vi "DataToVAttrbutes.vi"(6 "to lowercase?(T)":bool=TRUE, 8 "error in (no error)":errorcluster, 11 "data":variant) -> (0 "error out":errorcluster, 3 "VAttributes":variant)   [LabVIEW 2019]
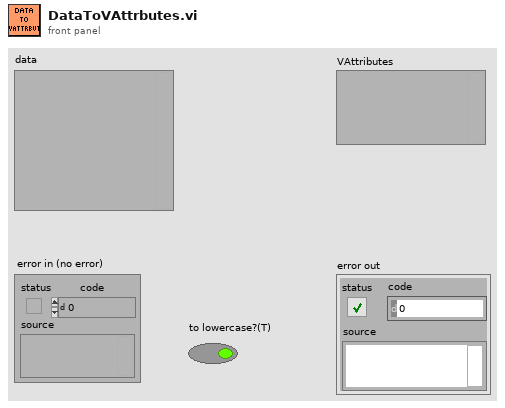
[diagram p1: front panel]
types:
  T1 = typedef "Type Descriptor Enumeration__ogtk.ctl" = enum8{"<Null>", "I8", "I16", "I32", "I64", "U8", "U16", "U32", "U64", "SGL", "DBL", "EXT", "CSG", "CDB", "CXT", "0x0F", "0x10", "0x11", "0x12", "0x13", "0x14", "Enum U8", "Enum U16", "Enum U32", "Enum U64", "SGL PQ", "DBL PQ", "EXT PQ", "CSG PQ", "CDB PQ", "CXT PQ", "0x1F", "0x20", "Boolean", "0x22", "0x23", "0x24", "0x25", "0x26", "0x27", "0x28", "0x29", "0x2A", "0x2B", "0x2C", "0x2D", "0x2E", "0x2F", "String", "0x31", "Path", "Pict", "0x34", "0x35", "0x36", "DAQ", "0x38", "0x39", "0x3A", "0x3B", "0x3C", "0x3D", "0x3E", "0x3F", "Array", "0x41", "0x42", "0x43", "0x44", "0x45", "0x46", "0x47", "0x48", "0x49", "0x4A", "0x4B", "0x4C", "0x4D", "0x4E", "0x4F", "Cluster", "0x51", "0x52", "Variant", "Waveform", "0x55", "0x56", "0x57", "0x58", "0x59", "0x5A", "0x5B", "0x5C", "0x5D", "0x5E", "0x5F", "0x60", "0x61", "0x62", "0x63", "0x64", "0x65", "0x66", "0x67", "0x68", "0x69", "0x6A", "0x6B", "0x6C", "0x6D", "0x6E", "0x6F", "Refnum"}
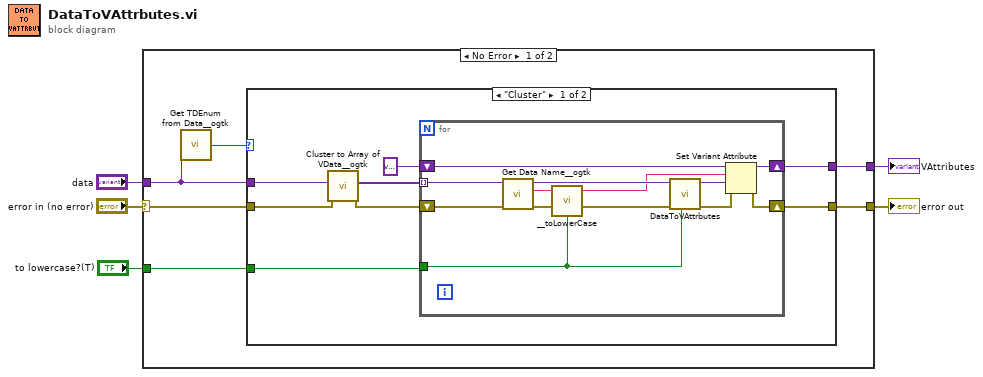
[diagram p0: block diagram]
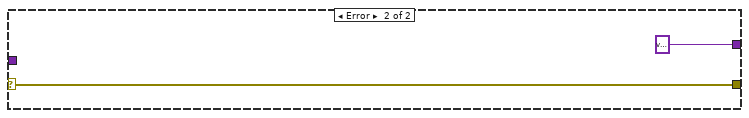
[diagram p3: hidden frame]
diagram:
  n1 = case shown="No Error" "error in (no error)" {
    selector: "error in (no error)" -> [w8 w35]
    tunnel: "data" -> [w11 _]
    tunnel: [w10 variant ("variant")] -> w4
    tunnel: [w9 w35] -> w3
    tunnel: "to lowercase?(T)" -> [w7 _]
    frame No Error {
      n2 = call <userlib>:"Get TDEnum from Data__ogtk.vi"("Data"=w11) -> ("Type Descriptor Enumeration"=w6:T1)  [unwired: 4 in]
      n3 = case shown="\"Cluster\"" w6 {
        tunnel: w11 -> [w19 w32]
        tunnel: [w18 w32] -> w10
        tunnel: [w17 w33] -> w9
        tunnel: w8 -> [w16 w33]
        tunnel: w7 -> [w15 _]
        frame "Cluster" {
          n4 = call <userlib>:"Cluster to Array of VData__ogtk.vi"("error in (no error)"=w16, "Cluster"=w19) -> ("error out"=w12:errorcluster, "Array of VData"=w14:variant[])  [unwired: 8 in]
          n5 = for {
            tunnel: w14 -> [w31] mode=indexing
            shift-right: [w28] -> w18
            shift-left: variant ("variant") -> [w29]
            shift-right: [w22] -> w17
            shift-left: w12 -> [w23]
            tunnel: w15 -> [w20]
            n6 = call <userlib>:"Get Data Name__ogtk.vi"("error in (no error)"=w23, "Data"=w31) -> ("error out"=w24:errorcluster, "Data Name"=w30:string, "Data dup"=w27:variant)  [unwired: 7 in]
            n7 = call "__toLowerCase.vi"("Data Name in"=w30, "to lowercase?(F)"=w20) -> ("Data Name out"=w21:string)  [unwired: 5 in]
            n8 = call "DataToVAttrbutes.vi"("to lowercase?(T)"=w20, "error in (no error)"=w24, "data"=w27) -> ("error out"=w25:errorcluster, "VAttributes"=w26:variant)  [unwired: 7 in]
            n9 = Set Variant Attribute(Variant=w29, name=w21, value=w26, error in=w25) -> (Variant out=w28:variant, error out=w22:errorcluster)  [unwired: 1 out]
          }
        }
        frame Default {
        }
      }
    }
    frame Error {
    }
  }
  "VAttributes" <- w4
  "error out" <- w3
